vi "QT_SoundToWaveform.vi"(7 "Sound in":T1 {"Rate" format="%x"}) -> (4 "mono 16-bit":i16[](array[numeric]), 6 "mono 8-bit":u8[](array[numeric]), 8 "sound format":T2, 10 "stereo 8-bit":u8[][](array[numeric]), 13 "display":i16[][](array[numeric]), 15 "stereo 16-bit":i16[][](array[numeric]))   [LabVIEW 2024]
uses:
  <vilib>/sound/lvsound.llb/Sound Format.ctl
  <userlib>/ImageProcessing/QTLIB_2595_LV86/QT_Sound.ctl
panel:
  out "Waveform Chart":i16[][](graph)
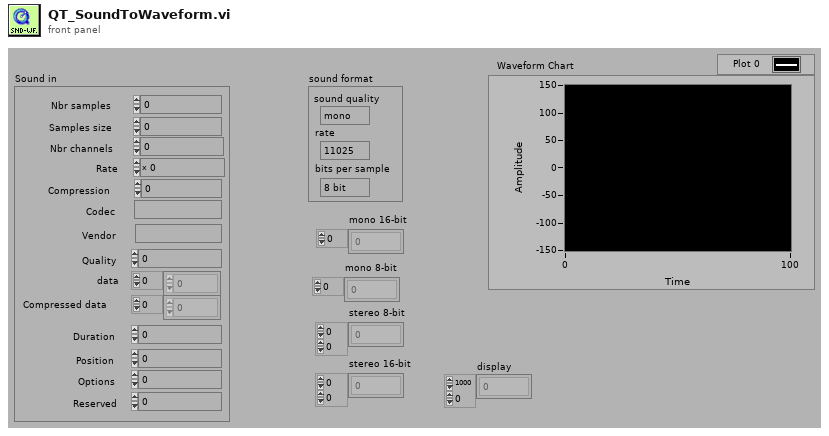
[diagram p1: front panel]
types:
  T1 = typedef "QT_Sound.ctl" = cluster{"Nbr samples":i32, "Samples size":i32, "Nbr channels":i32, "Rate ":i32, "Compression":i32, "Codec":string, "Vendor":string, "Quality":i32, "data":i16[], "Compressed data":u8[], "Duration":i32, "Position":i32, "Options":i32, "Reserved":i32}
  T2 = typedef "Sound Format.ctl" = cluster{"sound quality":enum16{"mono", "stereo"}, "rate":enum16{"11025", "22050", "44100", "8000"}, "bits per sample":enum16{"8 bit", "16 bit"}}
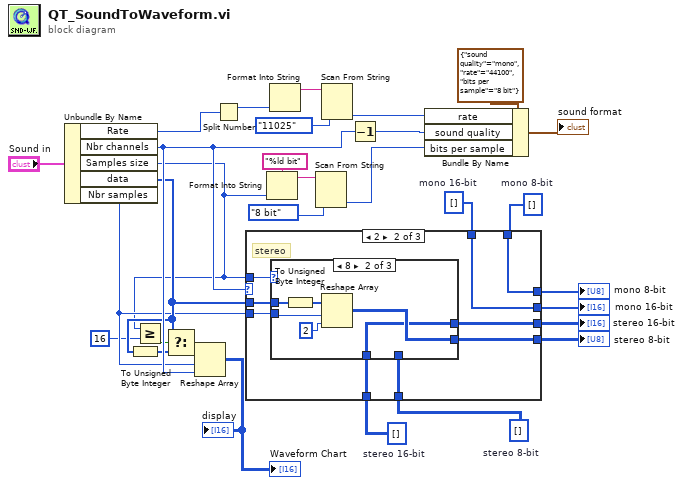
[diagram p0: block diagram]
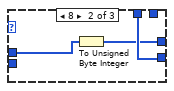
[diagram p3: hidden frame]
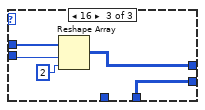
[diagram p6: hidden frame]
diagram:
  w14 = u8[][] []  # stereo 8-bit
  w13 = i16[][] []  # stereo 16-bit
  w15 = i16[] []  # mono 16-bit
  w16 = u8[] []  # mono 8-bit
  n1 = Unbundle By Name("Sound in") -> ("Rate"=w2:i32, "Nbr channels"=w11:i32, "Samples size"=w3:i32, "data"=w8:i16[], "Nbr samples"=w6:i32)
  n2 = To Unsigned Byte Integer(number=w8) -> (unsigned 8bit integer=w9:u8[])
  n3 = Greater Or Equal?(x=w3, y=16) -> (x >= y?=w5:bool)
  n4 = Select(t=w8, s=w5, f=w9) -> (s? t:f=w7:i16[])
  n5 = Reshape Array(w7, w6, w11) -> (→"display" →"Waveform Chart":i16[][])
  n6 = Split Number(x=w2) -> (hi(x)=w1:u16)  [unwired: 1 out]
  n7 = case shown="2" w11 {
    tunnel: w6 -> [w39 w55 _]
    tunnel: w8 -> [w38 w54 _]
    tunnel: w3 -> [w37 w53 _]
    tunnel: [w36 w48 w72] -> w20
    tunnel: [w34 w49 w70] -> w19
    tunnel: [w32 w47 w71] -> w18
    tunnel: [w35 w50 w69] -> w17
    tunnel: w16 -> [w31 w48 w72]
    tunnel: w15 -> [w33 w47 w71]
    tunnel: w14 -> [w34 w51 w70]
    tunnel: w13 -> [w35 w52 w69]
    frame 1 {
      # "mono"
      n8 = case shown="0, Default" w37 {
        tunnel: w39 -> [_ _ _]
        tunnel: w38 -> [_ w44 w45]
        tunnel: [w40 w42 w46] -> w36
        tunnel: [w41 w43 w45] -> w32
        tunnel: w33 -> [w41 w43 _]
        tunnel: w31 -> [w40 _ w46]
        frame 0, Default {
        }
        frame 8 {
          n9 = To Unsigned Byte Integer(number=w44) -> (unsigned 8bit integer=w42:u8[])
        }
        frame 16 {
        }
      }
    }
    frame 2 {
      # "stereo"
      n10 = case shown="8" w53 {
        tunnel: w55 -> [_ w62 w66]
        tunnel: w54 -> [_ w63 w67]
        tunnel: [w57 w60 w68] -> w49
        tunnel: w52 -> [w56 w59 _]
        tunnel: w51 -> [w57 _ w68]
        tunnel: [w56 w59 w64] -> w50
        frame 0, Default {
        }
        frame 8 {
          n11 = To Unsigned Byte Integer(number=w63) -> (unsigned 8bit integer=w58:u8[])
          n12 = Reshape Array(w58, w62, 2 ("dimension size")) -> (w60:u8[][])
        }
        frame 16 {
          n13 = Reshape Array(w67, w66, 2 ("dimension size")) -> (w64:i16[][])
        }
      }
    }
    frame 0, Default {
    }
  }
  "mono 8-bit" <- w20
  "mono 16-bit" <- w18
  "stereo 16-bit" <- w17
  "stereo 8-bit" <- w19
  n14 = Format Into String(format string="%ld bit", w3) -> (resulting string=w27:string)  [unwired: 2 in, 1 out]
  n15 = Format Into String(w1) -> (resulting string=w26:string)  [unwired: 3 in, 1 out]
  n16 = Scan From String(input string=w27, default 1=enum16{"8 bit", "16 bit"}."8 bit" ("bits per sample")) -> (output 1=w29:enum16{"8 bit", "16 bit"})  [unwired: 3 in, 3 out]
  n17 = Scan From String(input string=w26, default 1=enum16{"11025", "22050", "44100", "8000"}."11025" ("rate")) -> (output 1=w21:enum16{"11025", "22050", "44100", "8000"})  [unwired: 3 in, 3 out]
  n18 = Decrement(x=w11) -> (x-1=w12:i32)
  n19 = Bundle By Name(cluster=T2 {"sound quality"=enum."mono", "rate"=enum."44100", "bits per sample"=enum."8 bit"} ("sound format"), "rate"=w21, "sound quality"=w12, "bits per sample"=w29) -> (→"sound format":T2)
